vi "Draw a Limbus Circle.vi"(7 "Img In":T2, 9 "IP Results":T1, 11 "Img Dest":T2) -> (2 "output cluster":T3, 3 "Img Out":T2(plugin-control))   [LabVIEW 2015]
uses:
  <vilib>/vision/Image Controls.llb/IMAQ Image.ctl
  IP results.ctl
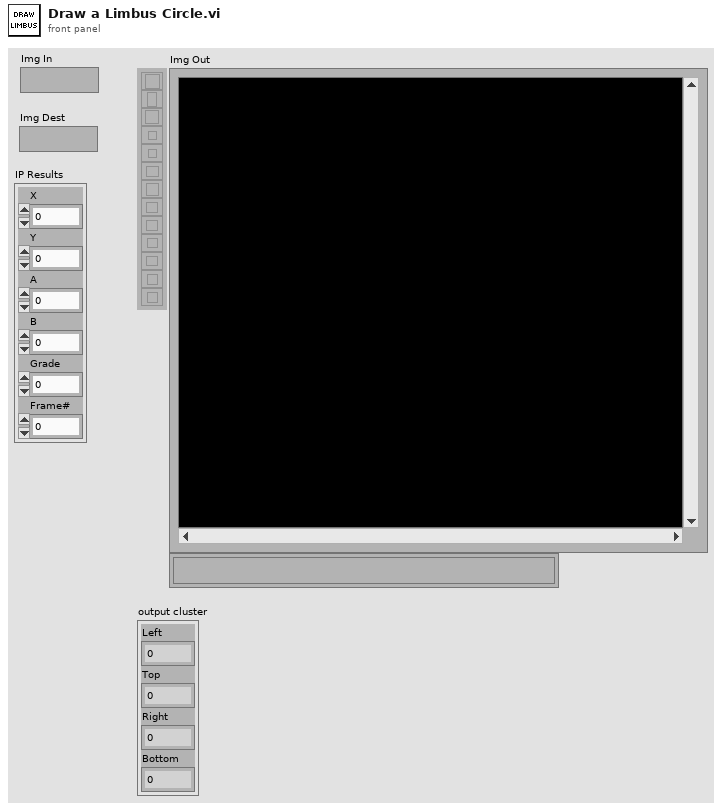
[diagram p1: front panel]
types:
  T1 = typedef "IP results.ctl" = cluster{"X":u16, "Y":u16, "A":dbl, "B":dbl, "Grade":u16, "Frame#":u16}
  T2 = typedef "IMAQ Image.ctl" = refnum<image>
  T3 = cluster{"Left":i32, "Top":i32, "Right":i32, "Bottom":i32}
  T4 = cluster{"Left":dbl, "Top":dbl, "Right":dbl, "Bottom":dbl}
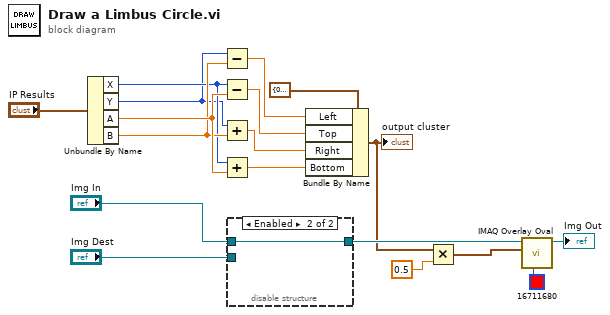
[diagram p0: block diagram]
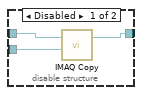
[diagram p2: hidden frame]
diagram:
  n1 = Unbundle By Name("IP Results") -> ("X"=w5:u16, "Y"=w4:u16, "A"=w7:dbl, "B"=w6:dbl)
  n2 = Subtract(x=w4, y=w6) -> (x-y=w10:dbl)
  n3 = Subtract(x=w5, y=w7) -> (x-y=w12:dbl)
  n4 = Add(x=w4, y=w6) -> (x+y=w11:dbl)
  n5 = Add(x=w5, y=w7) -> (x+y=w13:dbl)
  n6 = disable-structure shown="Enabled" {
    disable-tunnel: "Img In" -> [w21 w22]
    disable-tunnel: [w20 w22] -> w15
    disable-tunnel: "Img Dest" -> [w19 _]
    frame Disabled {
      n7 = call "IMAQ Copy"("Image Dst"=w19, "Image Src"=w21) -> ("Image Dst Out"=w20:T2)  [unwired: 1 in, 4 out]
    }
    frame Enabled {
    }
  }
  n8 = Bundle By Name(cluster=T3 {"Left"=0, "Top"=0, "Right"=0, "Bottom"=0} ("Bounding Rectangle"), "Left"=w10, "Top"=w12, "Right"=w11, "Bottom"=w13) -> (w3:T3)
  "output cluster" <- w3
  n9 = Multiply(x=w3, y=0.5) -> (x*y=w2:T4)
  n10 = call "IMAQ Overlay Oval"("Color"=u32 16711680, "Bounding Rectangle"=w2, "Image"=w15) -> ("Image Out"=→"Img Out":T2)  [unwired: 7 in, 1 out]
